vi "Fetch Library Methods Info.vi"(5 "Parser Settings":T9, 8 "Error in":errorcluster caption="Error in (no error)", 11 "Library in":refnum<vi>) -> (0 "Error out":errorcluster, 2 "Methods":T1[](array[typedef]))   [LabVIEW 2023, in "VIDoc Parsing.lvlib" / "Library Documentation.lvclass"]
doc: "Fetches the Library's Method information"
uses:
  Library Documentation.lvclass
  Settings/Parser Settings/Parser Settings Cluster.ctl
  Settings/Parser Settings/Draw Controls Cluster.ctl
  Settings/Parser Settings/Draw Option Enum.ctl
  TypeDefs/Method Spec Cluster.ctl
  TypeDefs/VI Type Extended Enum.ctl
  <vilib>/picture/picture.llb/imagedata.ctl
  TypeDefs/Class Dispatch Type Enum.ctl
  TypeDefs/Controls Info Cluster.ctl
  <vilib>/Utility/miscctls.llb/LVKeyTypeDef.ctl
  <vilib>/Utility/miscctls.llb/LVPointTypeDef.ctl
  SubVIs/Structure Reporter/Tree Cluster.ctl
  Library Documentation.lvclass/Library Documentation.ctl
  VIDoc Parsing.lvlib
  Settings/Parser Settings/Parser Settings.lvclass
  SubVIs/Structure Reporter/Structure Reporter.lvlib
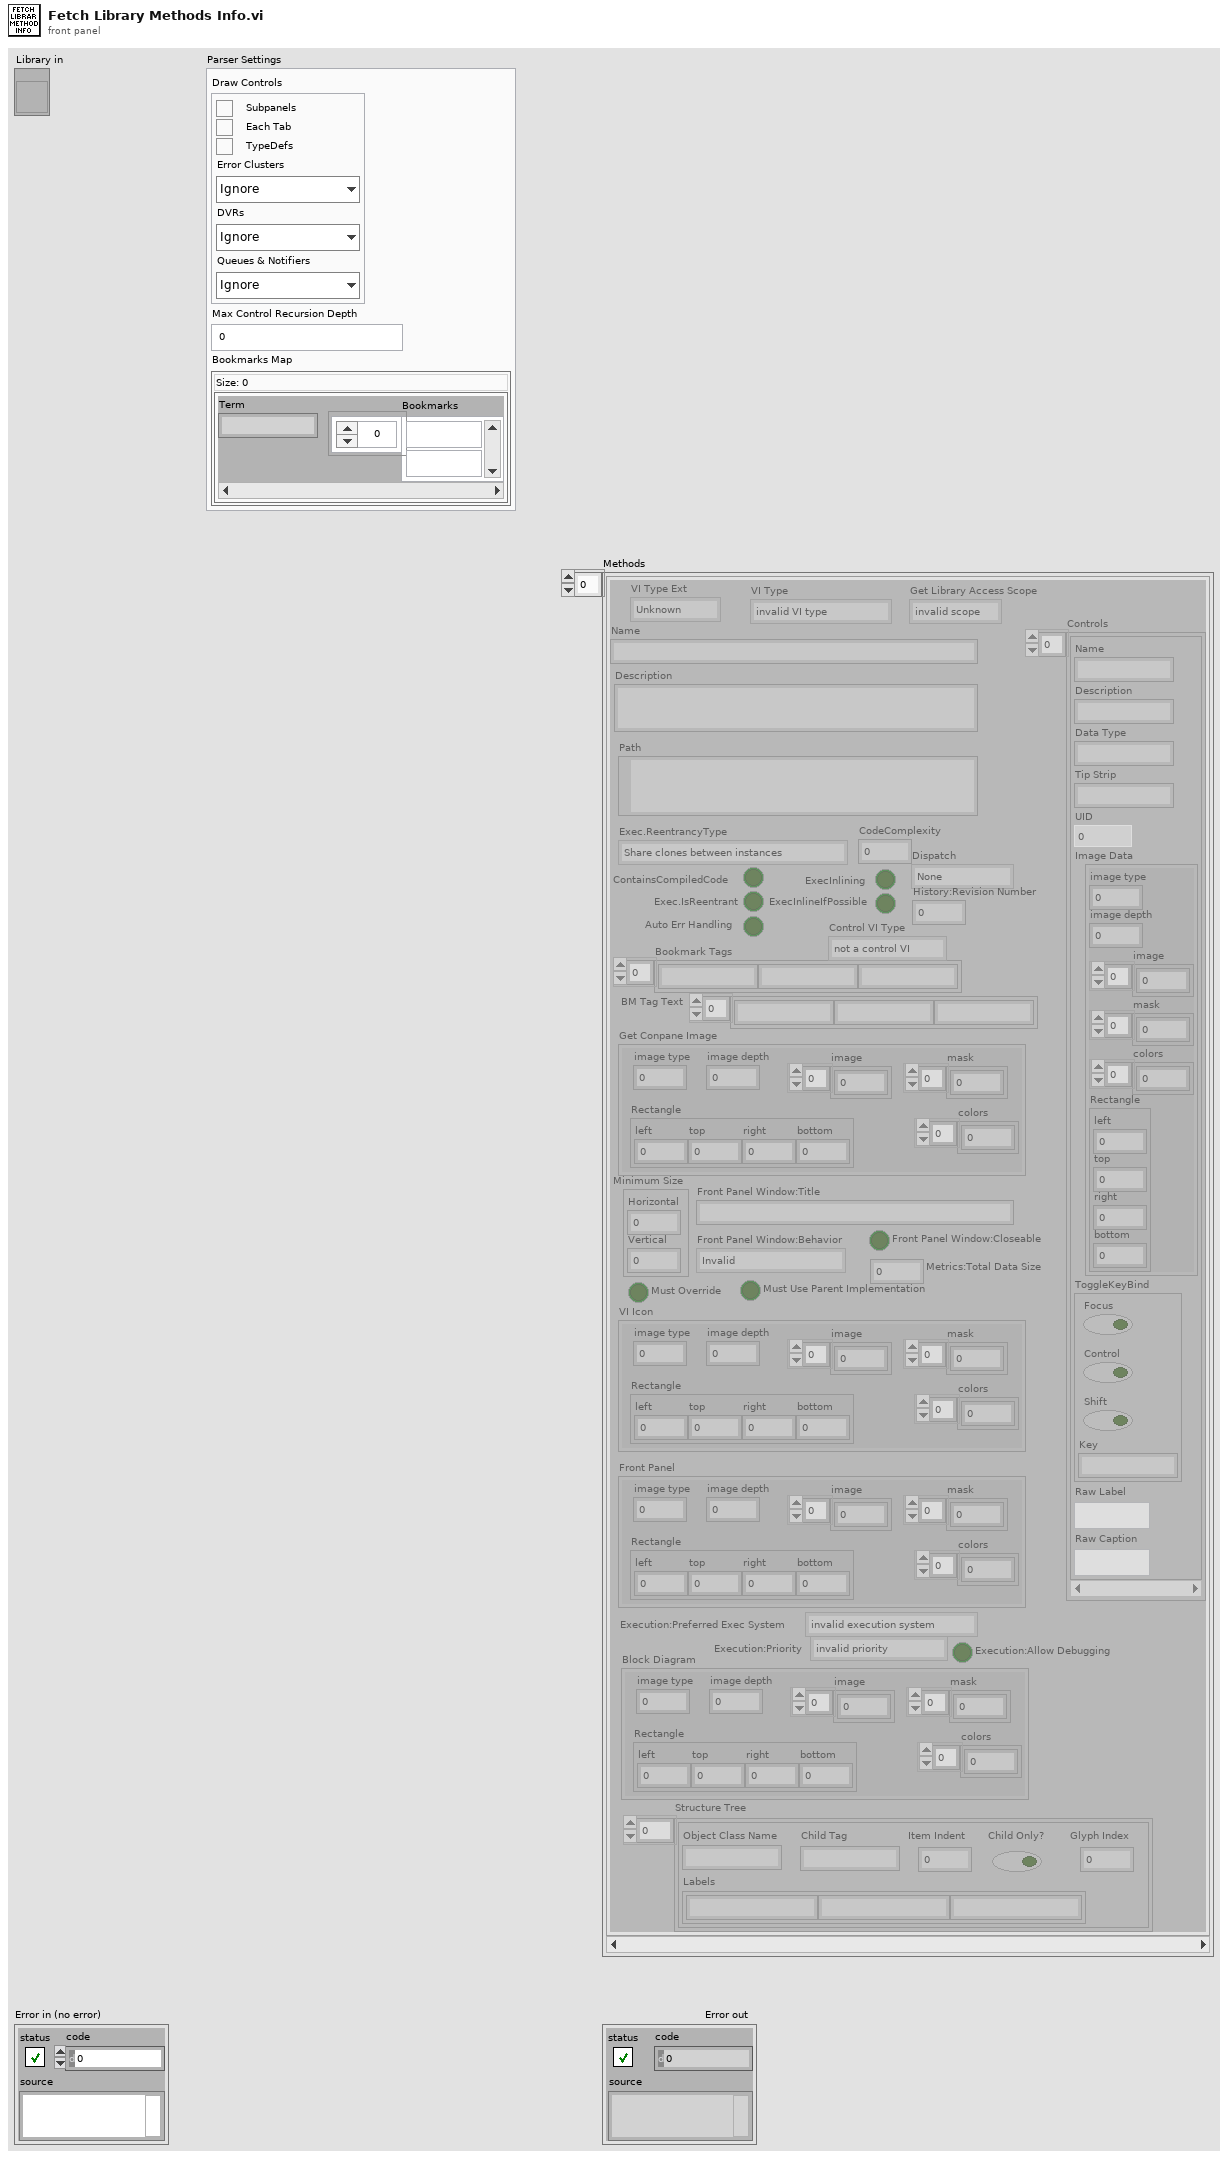
[diagram p1: front panel]
types:
  T1 = typedef "VIDoc Parsing.lvlib/Method Spec Cluster.ctl" = cluster{"VI Type Ext":T2, "Name":string, "Path":path, "Get Conpane Image":T3, "Description":string, "Get Library Access Scope":enum32{"invalid scope", "public", "private", "protected", "community"}, "Dispatch":T4, "ContainsCompiledCode":bool, "Exec.IsReentrant":bool, "Exec.ReentrancyType":enum16{"Share clones between instances", "Preallocate clone for each instance"}, "ExecInlining":bool, "ExecInlineIfPossible":bool, "Auto Err Handling":bool, "CodeComplexity":sgl, "Bookmark Tags":string[], "Control VI Type":enum32{"not a control VI", "control", "typedef", "strict typedef"}, "Controls":T5[], "VI Type":enum32{"invalid VI type", "Standard VI", "Control VI", "Global VI", "Polymorphic VI", "Configuration VI", "SubSystem", "Facade VI", "Method VI", "Statechart Diagram VI"}, "Minimum Size":T7, "Front Panel Window:Title":string, "Front Panel Window:Behavior":enum32{"Invalid", "Default", "Floating", "Floating/Auto-Hide", "Modal"}, "Front Panel Window:Closeable":bool, "Must Override":bool, "Must Use Parent Implementation":bool, "VI Icon":T3, "Front Panel":T3, "History:Revision Number":u32, "Metrics:Total Data Size":u32, "Execution:Allow Debugging":bool, "Execution:Preferred Exec System":enum32{"invalid execution system", "user interface", "standard", "instrument i/o", "data acquisition", "other 1", "other 2", "same as caller"}, "Execution:Priority":enum32{"invalid priority", "background priority", "normal priority", "above normal priority", "high priority", "time critical priority", "subroutine"}, "BM Tag Text":string[], "Block Diagram":T3, "Structure Tree":T8[]}
  T2 = typedef "VIDoc Parsing.lvlib/VI Type Extended Enum.ctl" = enum16{"Unknown", "Class Method", "Class Accessor Get", "Class Accessor Set", "Class Control", "Library Method", "Library Control", "VI", "Control"}
  T3 = typedef "imagedata.ctl" = cluster{"image type":i32, "image depth":i32, "image":u8[], "mask":u8[], "colors":u32[], "Rectangle":cluster{"left":i16, "top":i16, "right":i16, "bottom":i16}}
  T4 = typedef "VIDoc Parsing.lvlib/Class Dispatch Type Enum.ctl" = enum16{"None", "Static", "Dynamic"}
  T5 = typedef "VIDoc Parsing.lvlib/Controls Info Cluster.ctl" = cluster{"Name":string, "Description":string, "Data Type":string, "Tip Strip":string, "UID":i32, "Image Data":T3, "ToggleKeyBind":T6, "Raw Label":string, "Raw Caption":string}
  T6 = typedef "LVKeyTypeDef.ctl" = cluster{"Focus":bool, "Control":bool, "Shift":bool, "Key":string}
  T7 = typedef "LVPointTypeDef.ctl" = cluster{"Horizontal":i16, "Vertical":i16}
  T8 = typedef "VIDoc Parsing.lvlib/Structure Reporter.lvlib/Tree Cluster.ctl" = cluster{"Object Class Name":string, "Labels":string[], "Child Tag":string, "Item Indent":i32, "Child Only?":bool, "Glyph Index":i32}
  T9 = typedef "VIDoc Parsing.lvlib/Parser Settings.lvclass/Parser Settings Cluster.ctl" = cluster{"Draw Controls":T10, "Max Control Recursion Depth":i32, "Bookmarks Map":map{string, string[]}}
  T10 = typedef "VIDoc Parsing.lvlib/Parser Settings.lvclass/Draw Controls Cluster.ctl" = cluster{"Subpanels":bool, "Tabs":bool, "TypeDefs":bool, "Error Clusters":T11, "DVRs":T11, "Queues & Notifiers":T11}
  T11 = typedef "VIDoc Parsing.lvlib/Parser Settings.lvclass/Draw Option Enum.ctl" = enum16{"Ignore", "Draw", "Draw + Contents"}
  T12 = enum32{"invalid VI type", "Standard VI", "Control VI", "Global VI", "Polymorphic VI", "Configuration VI", "SubSystem", "Facade VI", "Method VI", "Statechart Diagram VI"}
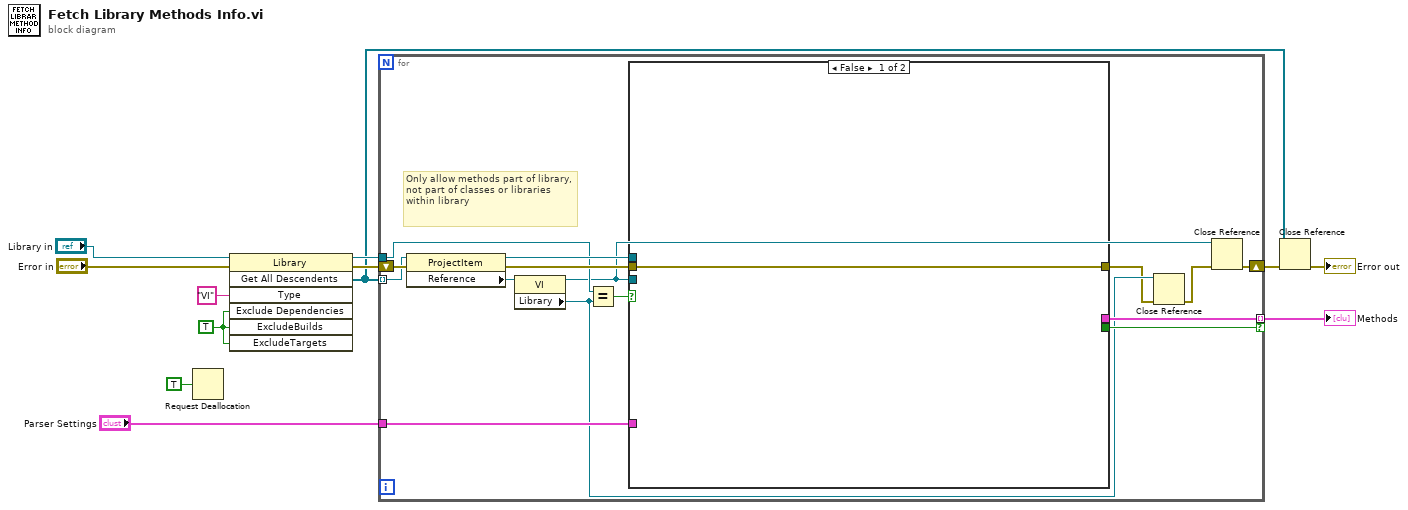
[diagram p0: block diagram]
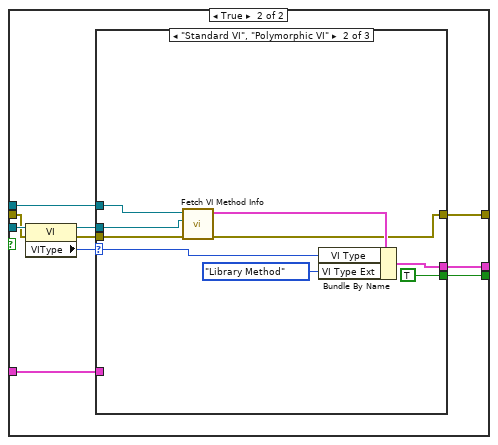
[diagram p2: hidden frame]
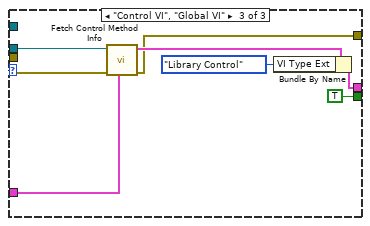
[diagram p4: hidden frame]
diagram:
  w10 = TRUE ("ExcludeDependencies")
  n1 = Request Deallocation(TRUE ("flag")) -> ()
  n2 = invoke class="Library" method="Get All Descendents"(reference="Library in", error in="Error in", "Type"="VI", "Exclude Dependencies"=w10, "ExcludeBuilds"=w10, "ExcludeTargets"=w10) -> (reference out=w9:refnum<vi>, error out=w7:errorcluster, "All Descendents"=w1:refnum<vi>[])  [unwired: 1 in, 4 out]
  n3 = for {
    tunnel: [w27] -> w8 mode=indexing if=w26
    tunnel: w9 -> [w18]
    tunnel: w1 -> [w20] mode=indexing
    shift-right: [w17] -> w3
    shift-left: w7 -> [w24]
    tunnel: "Parser Settings" -> [w22]
    # "Only allow methods part of library, not part of classes or libraries within library"
    n4 = property class="ProjectItem"(reference=w20, error in=w24) -> (reference out=w25:refnum<vi>, error out=w23:errorcluster, "Reference"=w19:refnum<vi>)
    n5 = property class="VI"(reference=w19) -> (reference out=w16:refnum<vi>, "Library"=w15:refnum<vi>)  [unwired: 1 in, 1 out]
    n6 = Equal?(x=w18, y=w15) -> (x = y?=w21:bool)
    n7 = case shown="False" w21 {
      tunnel: [_ w36] -> w27
      tunnel: [_ w35] -> w26
      tunnel: w25 -> [_ w34]
      tunnel: w16 -> [_ w33]
      tunnel: w23 -> [w28 w32]
      tunnel: [w28 w30] -> w14
      tunnel: w22 -> [_ w29]
      frame False {
      }
      frame True {
        n8 = property class="VI"(reference=w33, error in=w32) -> (reference out=w37:refnum<vi>, error out=w31:errorcluster, "VIType"=w38:T12)
        n9 = case shown="\"Standard VI\", \"Polymorphic VI\"" w38 {
          selector: w38 -> [_ w47 _]
          tunnel: w37 -> [_ w40 w54]
          tunnel: w34 -> [_ w45 _]
          tunnel: [_ w46 w50] -> w36
          tunnel: [_ TRUE TRUE] -> w35
          tunnel: w31 -> [w39 w43 w53]
          tunnel: [w39 w42 w52] -> w30
          tunnel: w29 -> [_ _ w51]
          frame Default {
          }
          frame "Standard VI", "Polymorphic VI" {
            n10 = call "Fetch VI Method Info.vi"("Error in"=w43, "VI Reference"=w40, "VI ProjectItem in"=w45) -> ("Error out"=w42:errorcluster, "Method Spec Cluster"=w44:T1)  [unwired: 7 in]
            n11 = Bundle By Name(cluster=w44, "VI Type"=w47, "VI Type Ext"=VI_Type_Extended_Enum."Library Method") -> (w46:T1)
          }
          frame "Control VI", "Global VI" {
            n12 = call "Fetch Control Method Info.vi"("Parser Settings"=w51, "Error in"=w53, "VI in"=w54) -> ("Error out"=w52:errorcluster, "Method Spec Cluster"=w55:T1)  [unwired: 7 in]
            n13 = Bundle By Name(cluster=w55, "VI Type Ext"=VI_Type_Extended_Enum."Library Control") -> (w50:T1)
          }
        }
      }
    }
    n14 = Close Reference(reference=w15, error in (no error)=w14) -> (error out=w13:errorcluster)
    n15 = Close Reference(reference=w16, error in (no error)=w13) -> (error out=w17:errorcluster)
  }
  "Methods" <- w8
  n16 = Close Reference(reference=w1, error in (no error)=w3) -> (error out=→"Error out":errorcluster)
